vi "Constructor.vi"(8 "error in (no error)":errorcluster, 10 "Product_Ref":string, 11 "Board in":refnum<class "Board.lvclass">) -> (0 "error out":errorcluster, 3 "Board out":refnum<class "Board.lvclass">)   [LabVIEW 2025, in "SW License Manager.lvlib" / "Board.lvclass"]
uses:
  Board.lvclass
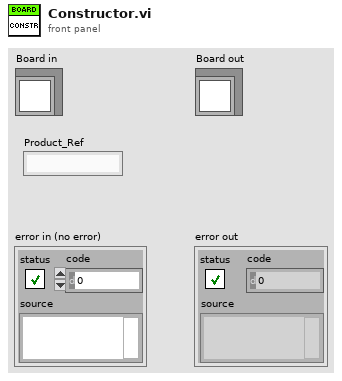
[diagram p1: front panel]
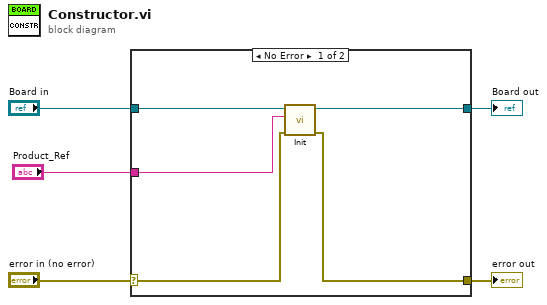
[diagram p0: block diagram]
diagram:
  n1 = case shown="No Error" "error in (no error)" {
    selector: "error in (no error)" -> [w8 w12]
    tunnel: [w7 w12] -> w4
    tunnel: [w9 w11] -> w2
    tunnel: "Board in" -> [w10 w11]
    tunnel: "Product_Ref" -> [w6 _]
    frame No Error {
      n2 = call-dynamic "Init.vi"("error in (no error)"=w8, "Product_Ref"=w6, "Board in"=w10) -> ("error out"=w7:errorcluster, "Board out"=w9:refnum<class "Board.lvclass">)  [unwired: 7 in]
    }
    frame Error {
    }
  }
  "error out" <- w4
  "Board out" <- w2
